vi "potenciometro.vi"() -> ()   [LabVIEW 2023]
uses:
  <vilib>/MakerHub/LINX/Public/Peripherals/Analog/Analog Read 1 Chan.vi
  <vilib>/MakerHub/LINX/Public/Peripherals/Analog/Analog Read N Chans.vi
  <vilib>/MakerHub/LINX/Private/Local IO/LinxAnalogRead.vi
  <vilib>/MakerHub/LINX/Public/Utilities/Check Channel.vi
  <vilib>/MakerHub/LINX/Public/Utilities/Open Serial.vi
  <vilib>/MakerHub/LINX/Private/Utilties/Generate Error.vi
  <vilib>/MakerHub/LINX/LMH-LINX.lvlib
panel:
  out "Loop Rate (Hz)":u32=5
  out "NS":dbl=51.0
  in  "tsim":dbl=10.0
  out "Ts":dbl=0.2
  in  "fs":dbl=5.0
  out "IT":i32=50
  out "Chart":dbl(graph)=0.869140625
  # "CON ESTO SE GENERA MI ARCHIVO data-pot.lvm"
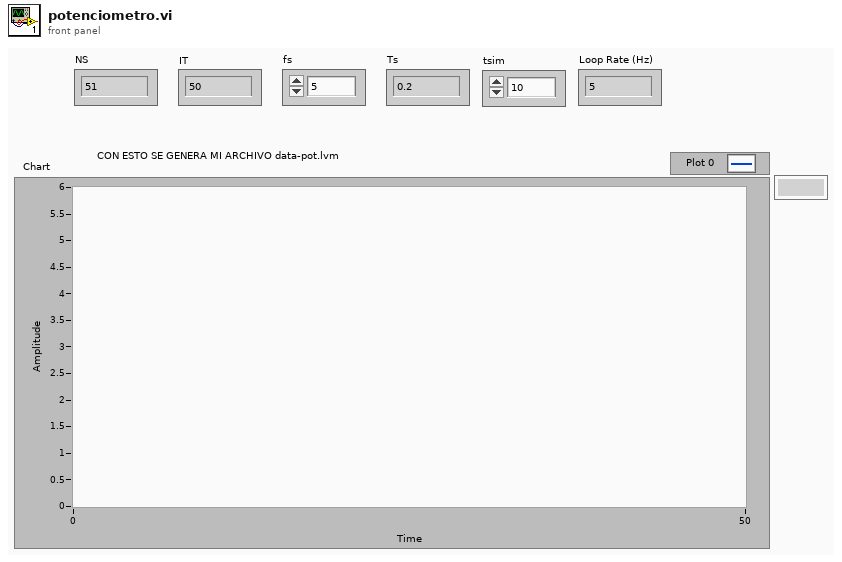
[diagram p1: front panel]
types:
  T1 = typedef "LMH-LINX.lvlib/LINX Ref.ctl" = cluster{"IO":T2, "Interface":T3, "LINX Device Config":T4}
  T2 = typedef "LMH-LINX.lvlib/Platform.ctl" = enum16{"Remote", "Local"}
  T3 = typedef "LMH-LINX.lvlib/Interface.ctl" = enum16{"Serial", "TCP"}
  T4 = typedef "LMH-LINX.lvlib/Device.lvlib/LINX Device Config.ctl" = cluster{"Interface":T3, "COM Port":refnum<visa-resource-name>, "TCP Configuration":T5, "Device Family":u8, "Device ID":u8, "Device Name":string, "TCP Ref":refnum<k5>, "Channels":T6}
  T5 = typedef "LMH-LINX.lvlib/Device.lvlib/TCP Config.ctl" = cluster{"IP Address":string, "Port":u16}
  T6 = typedef "LMH-LINX.lvlib/Channels.ctl" = cluster{"DI":u8[], "DO":u8[], "AI":u8[], "AO":u8[], "PWM":u8[], "QE":u8[], "UART":u8[], "I2C 2":u8[], "SPI":u8[], "CAN":u8[], "Servo":u8[], "AI Ref (V)":dbl, "AI Resolution (Bits)":u8, "AO Ref (V)":dbl, "AO Resolution (Bits)":u8}
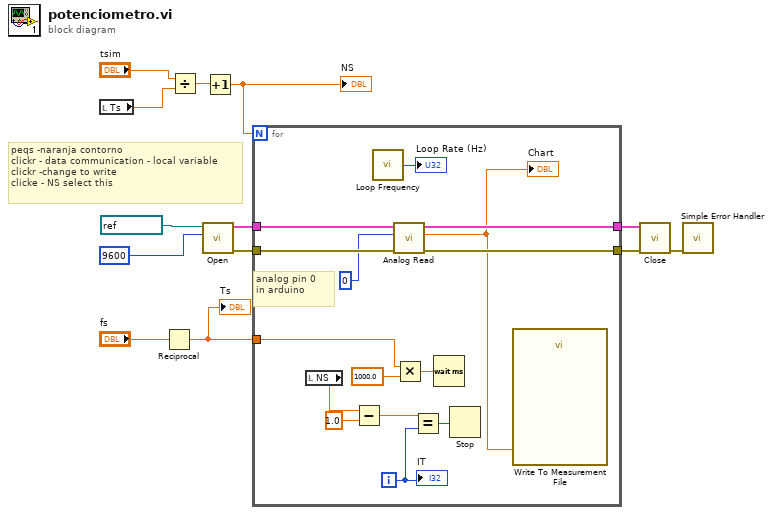
[diagram p0: block diagram]
diagram:
  # "peqs -naranja contorno \nclickr - data communication - local variable\nclickr -change to write\nclicke - NS select this"
  n1 = local read "Ts"() -> (w1:dbl)
  n2 = Reciprocal(x="fs") -> (1/x=w9:dbl)
  "Ts" <- w9
  n3 = Divide(x="tsim", y=w1) -> (x/y=w12:dbl)
  n4 = call-poly <vilib>:"Open.vi"("Baud Rate Override"=u32 9600, "Serial Port"=refnum<visa-resource-name> "COM7") -> ("Error Out"=w7:errorcluster, "LINX Resource"=w8:T1)  [unwired: 7 in, 1 out]
  n5 = Increment(x=w12) -> (x+1=w11:dbl)
  "NS" <- w11
  n6 = for {
    N: w11 -> [_]
    tunnel: w9 -> [w21]
    tunnel: w8 -> [w20]
    tunnel: w7 -> [w19]
    tunnel: [w18] -> w6
    tunnel: [w17] -> w5
    i -> [w26]
    # "analog pin 0 \nin arduino"
    n7 = local read "NS"() -> (w24:dbl)
    n8 = Subtract(x=w24, y=1.0) -> (x-y=w23:dbl)
    n9 = call <vilib>:"Loop Frequency.vi"() -> ("Loop Rate (Hz)"=→"Loop Rate (Hz)":u32)
    n10 = call-poly <vilib>:"Analog Read.vi"("Error In"=w19, "Analog Channel"=u8 0, "LINX Resource"=w20) -> ("Error Out"=w18:errorcluster, "Voltage"=w16:dbl, "LINX Resource"=w17:T1)  [unwired: 5 in, 1 out]
    "Chart" <- w16
    n11 = Multiply(x=w21, y=1000.0) -> (x*y=w28:dbl)
    n12 = Equal?(x=w23, y=w26) -> (x = y?=w22:bool)
    n13 = Wait (ms)(milliseconds to wait=w28) -> ()  [unwired: 1 out]
    n14 = Stop(stop? (T)=w22) -> ()
    n15 = call "Write To Measurement File"("Signals"=w16) -> ()  [unwired: 16 in, 3 out]
    "IT" <- w26
  }
  n16 = call <vilib>:"Close.vi"("Error In"=w6, "LINX Resource"=w5) -> ("Error Out"=w2:errorcluster)  [unwired: 9 in]
  n17 = call <vilib>:"Simple Error Handler.vi"("error in (no error)"=w2) -> ()  [unwired: 4 in, 5 out]
